vi "Write Allele-Bit.vi"(8 "error in (no error)":errorcluster, 10 "Allele-Bit":bool, 11 "IGene in":refnum<class "IGene.lvclass">) -> (0 "error out":errorcluster, 3 "IGene out":refnum<class "IGene.lvclass">)   [LabVIEW 2016, in "IGene.lvclass"]
uses:
  IGene.lvclass
  IGene.lvclass/IGene.ctl
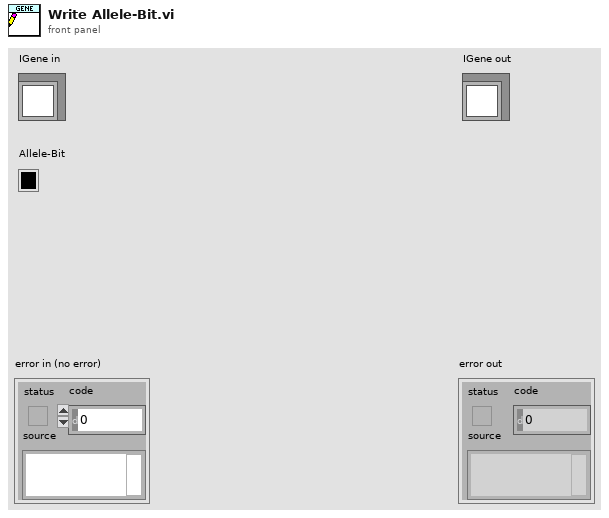
[diagram p1: front panel]
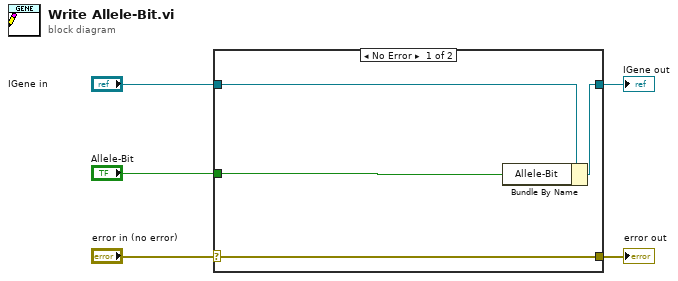
[diagram p0: block diagram]
diagram:
  n1 = case shown="No Error" "error in (no error)" {
    selector: "error in (no error)" -> [w9 w10]
    tunnel: [w9 w10] -> w4
    tunnel: [w7 w11] -> w2
    tunnel: "IGene in" -> [w8 w11]
    tunnel: "Allele-Bit" -> [w6 _]
    frame No Error {
      n2 = Bundle By Name(cluster=w8, "Allele-Bit"=w6) -> (w7:refnum<class "IGene.lvclass">)
    }
    frame Error {
    }
  }
  "error out" <- w4
  "IGene out" <- w2
